vi "Set.vi"(8 "error in (no error)":errorcluster, 10 "Numeric":dbl, 11 "Simulator in":refnum<class "Simulator.lvclass">) -> (0 "error out":errorcluster, 3 "Simulator out":refnum<class "Simulator.lvclass">)   [LabVIEW 2018, in "Simulator.lvclass"]
uses:
  Simulator.lvclass
  Simulator.lvclass/Simulator.ctl
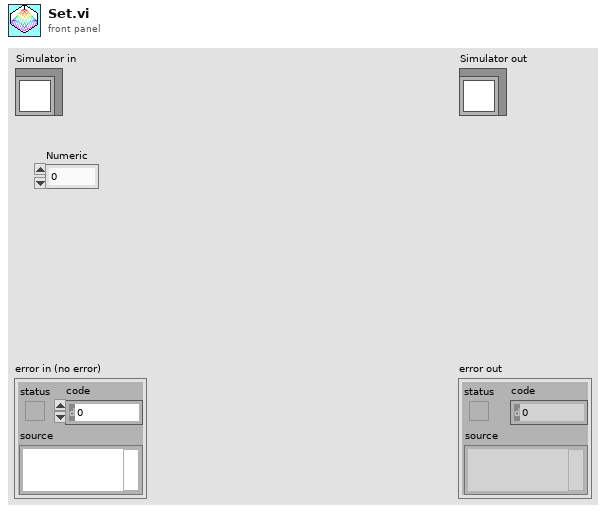
[diagram p1: front panel]
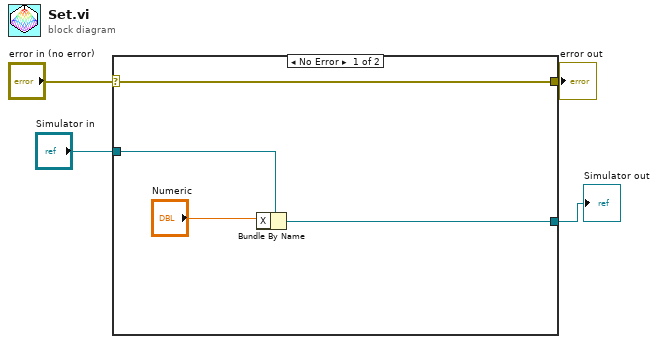
[diagram p0: block diagram]
diagram:
  n1 = case shown="No Error" "error in (no error)" {
    selector: "error in (no error)" -> [w8 w9]
    tunnel: [w8 w9] -> w3
    tunnel: "Simulator in" -> [w7 w10]
    tunnel: [w5 w10] -> w1
    frame No Error {
      n2 = Bundle By Name(cluster=w7, "X"="Numeric") -> (w5:refnum<class "Simulator.lvclass">)
    }
    frame Error {
    }
  }
  "error out" <- w3
  "Simulator out" <- w1
